vi "Double FFT Measurement Test UI.vi"() -> ()   [LabVIEW 2014]
uses:
  <vilib>/FPGAPlugInAG/sbRIO-9636/niLvFpga_Open_sbRIO-9636.vi
  <vilib>/rvi/interface/common/dynamic/niFpgaDynamicAddResources.vi
  <vilib>/rvi/interface/common/niFpgaWaitOnOcc.vi
  <vilib>/Utility/error.llb/Error Cluster From Error Code.vi
  <vilib>/rvi/errors/niLvFpgaAdjustHostInterfaceError.vi
  <vilib>/FPGAPlugInAG/Dynamic/niLvFpga_Close_Dynamic.vi
  <vilib>/rvi/interface/nirviOpenFPGA/nirviOpenFPGA.xnode
  FPGA Bitfiles/LaserDistanceSen_FPGATarget_DoubleFFTMeasure_H+-9Y7fLqeE.lvbitx
  FPGA Target/Test VIs/Double FFT Measurement (Init Memory) test.vi
  <vilib>/rvi/interface/nirviMethod/nirviMethod.xnode
  <vilib>/rvi/interface/nirviCloseFPGA/nirviCloseFPGA.xnode
  <vilib>/FPGAPlugInAG/Dynamic/niLvFpga_ConfigureFifo_Dynamic.vi
  <vilib>/rvi/errors/niLvFpgaMergeErrorWithErrorCode.vi
  <vilib>/FPGAPlugInAG/Dynamic/niLvFpga_StartFifo_Dynamic.vi
  <vilib>/FPGAPlugInAG/Dynamic/niLvFpga_ReadFifo_Dynamic.vi
  <vilib>/rvi/Analysis/host/Public/NI_FpgaMspHost.lvlib
panel:
  in  "Snapshot":bool
  in  "Sample Rate (S/s)":dbl=50000000.0 format="%#_13g"
  in  "l":T1(tab)
  out "Signal":waveform(dbl)(graph)
  out "Modulation Signal":waveform(dbl)(graph)
  out "FFT bin 1":dbl
  out "Detected Frequency (Hz)":dbl
  out "FFT 1":dbl[](graph)
  in  "#Samples":dbl=1024.0
  in  "#Periods":dbl=100.0
  out "Theoretical Freq.":dbl
  out "Error %":dbl
  out "Gen. Freq.":dbl=10000000.0 format="%#_13g"
  out "FFT2":dbl[](graph)
  out "FFT bin 2":dbl
  out "Detected Frequency (Hz) 2":dbl
  out "Modulation Signal S":waveform(dbl)(graph)
  out "Signal S":waveform(dbl)(graph)
  out "Detected Frequency (Hz) 2 S":dbl
  out "FFT bin 2 S":dbl
  out "FFT 2 S":dbl[](graph)
  out "FFT 1 S":dbl[](graph)
  out "Detected Frequency (Hz) 1 S":dbl
  out "FFT bin 1 S":dbl
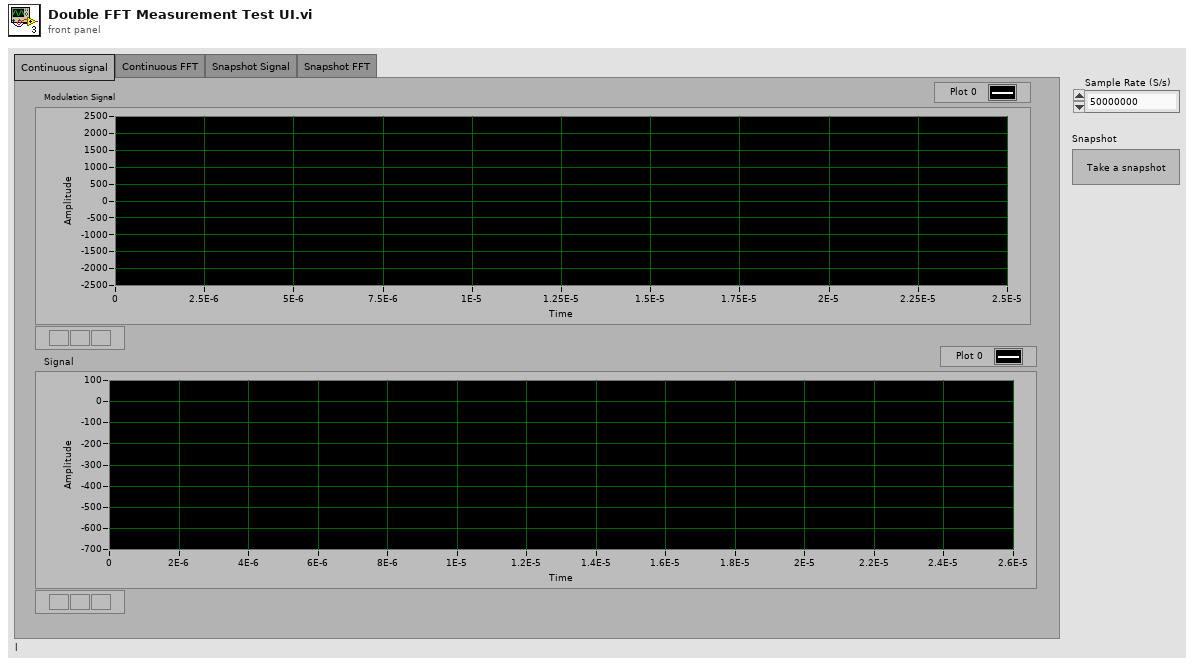
[diagram p1: front panel]
types:
  T1 = enum32{"Continuous signal", "Continuous FFT", "Snapshot Signal", "Snapshot FFT"}
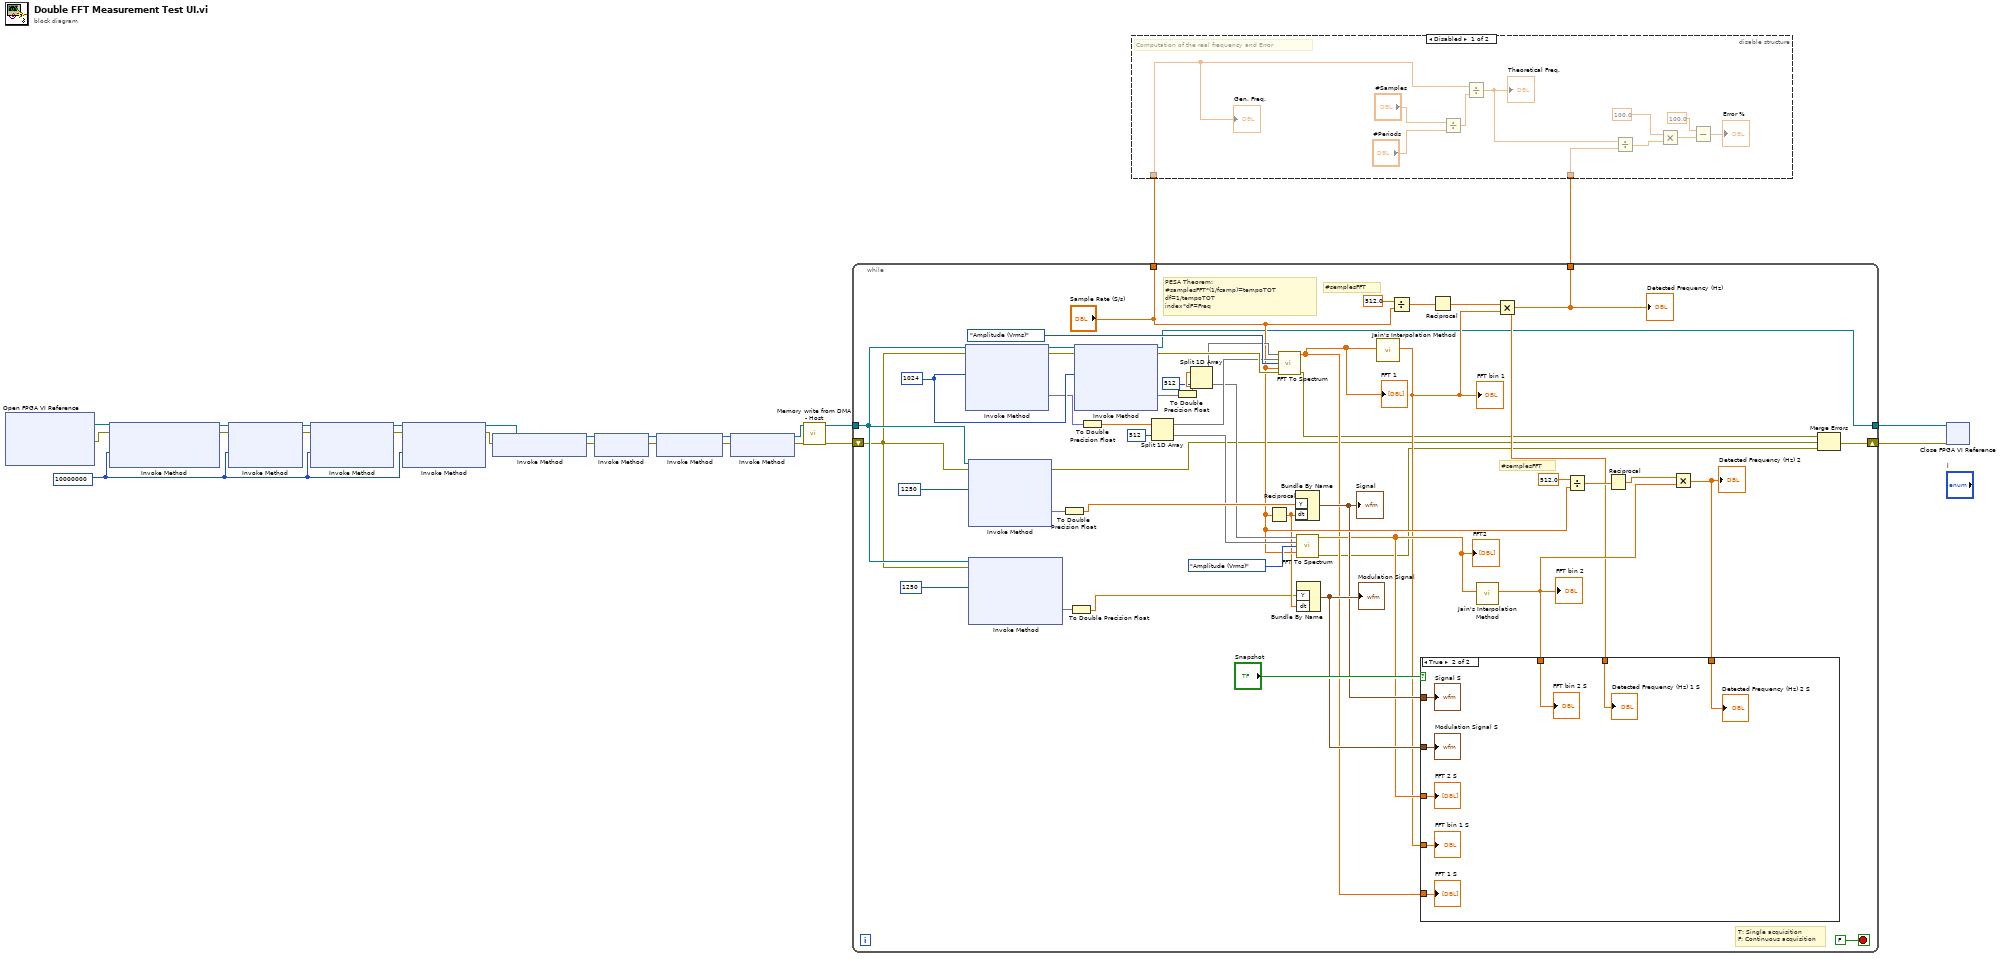
[diagram p0: block diagram]
diagram:
  w13 = u32 10000000 ("Requested Depth")
  n1 = xnode "Open FPGA VI Reference"() -> ("FPGA VI Reference Out"=w2:refnum<k20>, "error out"=w1:errorcluster)  [unwired: 2 in]
  n2 = xnode "Invoke Method"("FPGA VI Reference In"=w2, "error in"=w1, "Requested Depth"=w13) -> ("FPGA VI Reference Out"=w14:refnum<k20>, "error out"=w15:errorcluster)  [unwired: 1 out]
  n3 = xnode "Invoke Method"("FPGA VI Reference In"=w14, "error in"=w15, "Requested Depth"=w13) -> ("FPGA VI Reference Out"=w24:refnum<k20>, "error out"=w23:errorcluster)  [unwired: 1 out]
  n4 = xnode "Invoke Method"("FPGA VI Reference In"=w24, "error in"=w23, "Requested Depth"=w13) -> ("FPGA VI Reference Out"=w22:refnum<k20>, "error out"=w21:errorcluster)  [unwired: 1 out]
  n5 = xnode "Invoke Method"("FPGA VI Reference In"=w22, "error in"=w21, "Requested Depth"=w13) -> ("FPGA VI Reference Out"=w12:refnum<k20>, "error out"=w11:errorcluster)  [unwired: 1 out]
  n6 = xnode "Invoke Method"("FPGA VI Reference In"=w12, "error in"=w11) -> ("FPGA VI Reference Out"=w10:refnum<k20>, "error out"=w9:errorcluster)
  n7 = xnode "Invoke Method"("FPGA VI Reference In"=w10, "error in"=w9) -> ("FPGA VI Reference Out"=w20:refnum<k20>, "error out"=w19:errorcluster)
  n8 = xnode "Invoke Method"("FPGA VI Reference In"=w20, "error in"=w19) -> ("FPGA VI Reference Out"=w17:refnum<k20>, "error out"=w18:errorcluster)
  n9 = xnode "Invoke Method"("FPGA VI Reference In"=w17, "error in"=w18) -> ("FPGA VI Reference Out"=w4:refnum<k20>, "error out"=w3:errorcluster)
  n10 = call "Memory write from DMA - Host.vi"("error in"=w3, "FPGA VI Reference In"=w4) -> ("error out"=w5:errorcluster, "FPGA VI Reference Out"=w6:refnum<k20>)  [unwired: 6 in, 2 out]
  n11 = while {
    tunnel: [w35] -> w16
    tunnel: ["Sample Rate (S/s)"] -> w8
    shift-right: [w30] -> w7
    shift-left: w5 -> [w45]
    tunnel: w6 -> [w46]
    tunnel: [w29] -> w25
    stop <- FALSE stop-if-true
    w69 = u32 1024 ("Requested Depth")
    # "T: Single acquisition\nF: Continuous acquisition"
    # "PESA Theorem:\n#samplesFFT*(1/fcamp)=tempoTOT\ndf=1/tempoTOT\nindex*dF=Freq"
    # "#semplesFFT"
    # "#semplesFFT"
    n12 = xnode "Invoke Method"("FPGA VI Reference In"=w46, "error in"=w45, "Number of Elements"=w69) -> ("FPGA VI Reference Out"=w71:refnum<k20>, "error out"=w70:errorcluster, "Data"=w64:fxp<+/-,22,22>[])  [unwired: 1 in, 1 out]
    n13 = xnode "Invoke Method"("FPGA VI Reference In"=w46, "error in"=w45, "Number of Elements"=u32 1250) -> ("error out"=w32:errorcluster, "Data"=w68:fxp<+/-,12,12>[])  [unwired: 1 in, 2 out]
    n14 = xnode "Invoke Method"("FPGA VI Reference In"=w46, "error in"=w45, "Number of Elements"=u32 1250) -> ("Data"=w26:fxp<+/-,12,12>[])  [unwired: 1 in, 3 out]
    n15 = To Double Precision Float(number=w68) -> (double precision float=w67:dbl[])
    n16 = To Double Precision Float(number=w26) -> (double precision float=w43:dbl[])
    n17 = xnode "Invoke Method"("FPGA VI Reference In"=w71, "error in"=w70, "Number of Elements"=w69) -> ("FPGA VI Reference Out"=w29:refnum<k20>, "error out"=w66:errorcluster, "Data"=w65:fxp<+/-,22,22>[])  [unwired: 1 in, 1 out]
    n18 = To Double Precision Float(number=w64) -> (double precision float=w58:dbl[])
    n19 = Split 1D Array(array=w58, index=512) -> (second subarray=w53:dbl[])  [unwired: 1 out]
    n20 = To Double Precision Float(number=w65) -> (double precision float=w57:dbl[])
    n21 = Split 1D Array(array=w57, index=512) -> (first subarray=w55:dbl[], second subarray=w52:dbl[])
    n22 = Reciprocal(x="Sample Rate (S/s)") -> (1/x=w44:dbl)
    n23 = call <vilib>:"FFT To Spectrum.vi"("real FFT data"=w55, "imaginary FFT data"=w53, "spectrum type"=enum8{"Power (Vrms^2)", "Amplitude (Vrms)"}."Amplitude (Vrms)", "sample rate (S/s)"="Sample Rate (S/s)", "error in (no error)"=w66) -> ("spectrum out"=w36:dbl[], "error out"=w33:errorcluster)  [unwired: 8 in, 1 out]
    "FFT 1" <- w36
    n24 = Bundle By Name("Y"=w67, "dt"=w44) -> (w40:waveform(dbl))  [unwired: 1 in]
    "Signal" <- w40
    n25 = call <vilib>:"FFT To Spectrum.vi"("real FFT data"=w52, "imaginary FFT data"=w53, "spectrum type"=enum8{"Power (Vrms^2)", "Amplitude (Vrms)"}."Amplitude (Vrms)", "sample rate (S/s)"="Sample Rate (S/s)") -> ("spectrum out"=w39:dbl[], "error out"=w31:errorcluster)  [unwired: 9 in, 1 out]
    "FFT2" <- w39
    n26 = Bundle By Name("Y"=w43, "dt"=w44) -> (w41:waveform(dbl))  [unwired: 1 in]
    "Modulation Signal" <- w41
    n27 = call "Jain's Interpolation Method.vi"("FFT array"=w36) -> ("Index Bin"=w34:dbl)  [unwired: 9 in, 1 out]
    "FFT bin 1" <- w34
    n28 = Divide(x=512.0, y="Sample Rate (S/s)") -> (x/y=w61:dbl)
    n29 = Reciprocal(x=w61) -> (1/x=w60:dbl)
    n30 = call "Jain's Interpolation Method.vi"("FFT array"=w39) -> ("Index Bin"=w38:dbl)  [unwired: 9 in, 1 out]
    "FFT bin 2" <- w38
    n31 = Multiply(x=w60, y=w34) -> (x*y=w35:dbl)
    "Detected Frequency (Hz)" <- w35
    n32 = Divide(x=512.0, y="Sample Rate (S/s)") -> (x/y=w49:dbl)
    n33 = Reciprocal(x=w49) -> (1/x=w48:dbl)
    n34 = Multiply(x=w48, y=w38) -> (x*y=w37:dbl)
    "Detected Frequency (Hz) 2" <- w37
    n35 = case shown="True" "Snapshot" {
      tunnel: w41 -> [_ w79]
      tunnel: w40 -> [_ w78]
      tunnel: w39 -> [_ w77]
      tunnel: w38 -> [_ w76]
      tunnel: w37 -> [_ w75]
      tunnel: w36 -> [_ w74]
      tunnel: w35 -> [_ w72]
      tunnel: w34 -> [_ w73]
      frame False {
      }
      frame True {
        "FFT bin 2 S" <- w76
        "Detected Frequency (Hz) 1 S" <- w72
        "FFT bin 1 S" <- w73
        "Detected Frequency (Hz) 2 S" <- w75
        "Signal S" <- w78
        "FFT 1 S" <- w74
        "Modulation Signal S" <- w79
        "FFT 2 S" <- w77
      }
    }
    n36 = Merge Errors(w33, w32, w31) -> (w30:errorcluster)
  }
  n37 = disable-structure shown="Disabled" {
    disable-tunnel: w16 -> [w89 _]
    disable-tunnel: w8 -> [w80 _]
    frame Disabled {
      # "Computation of the real frequency and Error"
      n38 = Divide(x="#Samples", y="#Periods") -> (x/y=w90:dbl)
      n39 = Divide(x=w80, y=w90) -> (x/y=w88:dbl)
      "Theoretical Freq." <- w88
      n40 = Divide(x=w88, y=w89) -> (x/y=w87:dbl)
      n41 = Multiply(x=100.0, y=w87) -> (x*y=w83:dbl)
      n42 = Subtract(x=100.0, y=w83) -> (x-y=→"Error %":dbl)
      "Gen. Freq." <- w80
    }
    frame Enabled {
    }
  }
  n43 = xnode "Close FPGA VI Reference"("FPGA VI Reference In"=w25, "error in"=w7) -> ()  [unwired: 1 out]
